vi "Normalize(4D_SGL).vi"(7 "Norm Factor":sgl=400.0, 11 "Data In":sgl[][][](array[numeric])) -> (3 "Normalized Out":sgl[][][](array[numeric]))   [LabVIEW 2020]
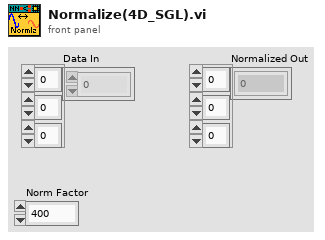
[diagram p1: front panel]
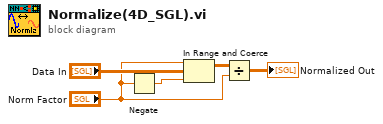
[diagram p0: block diagram]
diagram:
  n1 = Negate(x="Norm Factor") -> (-x=w1:sgl)
  n2 = In Range and Coerce(upper limit="Norm Factor", x="Data In", lower limit=w1) -> (coerced(x)=w5:sgl[][][])  [unwired: 1 out]
  n3 = Divide(x=w5, y="Norm Factor") -> (x/y=→"Normalized Out":sgl[][][])
